vi "GetI_MyINterface.vi"(0 "reference in":refnum<class "VdLaser.lvclass">, 5 "error in (no error)":errorcluster) -> (14 "reference out":refnum<class "VdLaser.lvclass">, 16 "InterfaceOut":refnum<class "MyINterface.lvclass">, 19 "error out":errorcluster)   [LabVIEW 2010, in "VdLaser.lvclass"]
doc: "Returns an Interaface that this class implements"
uses:
  VdLaser.lvclass
  MyINterface_Interface/MyINterface.lvclass
  VdLaser.lvclass/VdLaser.ctl
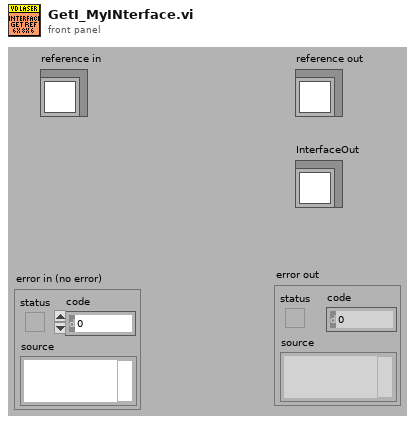
[diagram p1: front panel]
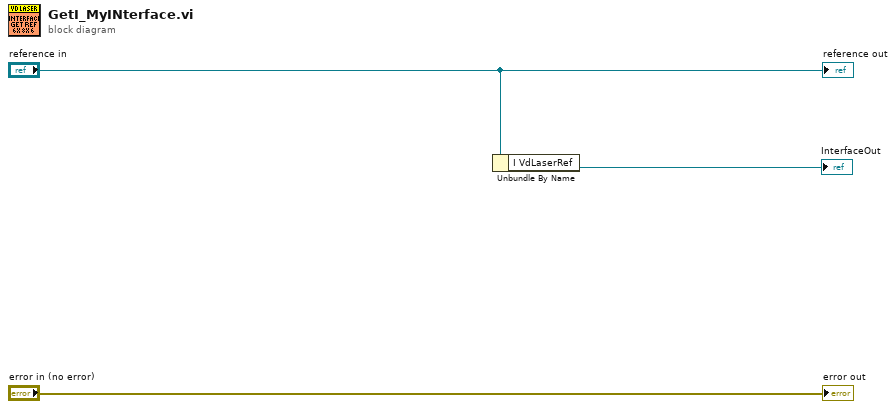
[diagram p0: block diagram]
diagram:
  n1 = Unbundle By Name("reference in") -> ("I VdLaserRef"=→"InterfaceOut":refnum<class "MyINterface.lvclass">)
  "error out" <- "error in (no error)"
  "reference out" <- "reference in"
